vi "Mcp2210 Request Spi Bus Rel.vi"(8 "error in (no error)":errorcluster, 10 "SPI Release ACK Pin Define":u8, 11 "handle":i32) -> (0 "error out":errorcluster, 3 "handle out":i32)   [LabVIEW 2015, in "mcp2210.lvlib"]
doc: "Request the release of the SPI bus and set the value of the \"SPI Bus Release ACK\" pin\nif GP7 is assigned to this dedicated function and if the bus can be released.\nIf SPI transfer is in progress, the bus is not released, the command returns M_E_ERR_SPI_XFER_ONGOING\nerrorcode and the host application should either wait the transfer completion or cancel it\n(by using M_Mcp2210_CancelSpiTxfer) and request again the SPI bus release.\nParameters:\nInputs:\n- IntPtr handle - The device handle. Cannot be NULL.\n- unsigned char ackPinVal - the value of the \"SPI Bus Release ACK\" pin if the\ncommand succeeds and the GP7 is assigned to alternate function 2.\nOutputs:\n- none\nReturns:\n- 0 for success: M_E_SUCCESS\n- negative error code: M_E_ERR_NULL, M_E_ERR_INVALID_HANDLE_VALUE, M_E_ERR_INVALID_PARAMETER\nM_E_ERR_UNKOWN_ERROR\nM_E_ERR_HID_TIMEOUT, M_E_ERR_HID_RW_FILEIO\nM_E_ERR_CMD_ECHO, M_E_ERR_CMD_FAILED\nM_E_ERR_SPI_XFER_ONGOING\n\nMCP2210_DLL_UM_API int __stdcall Mcp2210_RequestSpiBusRel(void *handle, unsigned char ackPinVal);"
uses:
  <userlib>/mcp2210/mcp2210.lvlib
  <userlib>/mcp2210/mcp2210_dll_um_x86.dll
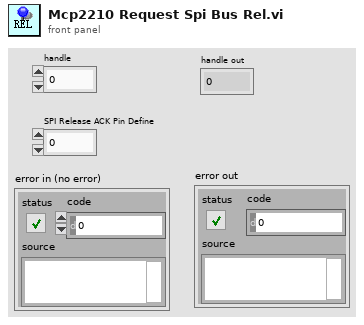
[diagram p1: front panel]
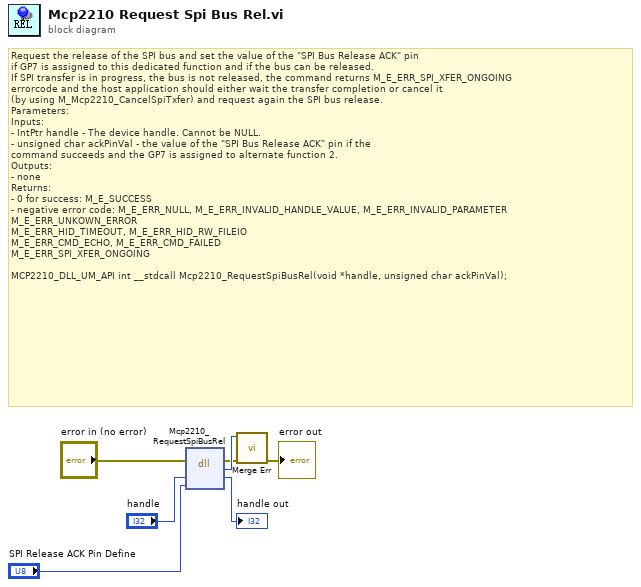
[diagram p0: block diagram]
diagram:
  # "Request the release of the SPI bus and set the value of the \"SPI Bus Release ACK\" pin\nif GP7 is assigned to this dedicated function and if the bus can be released.\nIf SPI transfer is in progress, the bus is not released, the command returns M_E_ERR_SPI_XFER_ONGOING\nerrorcode and the host application should either wait the transfer completion or cancel it\n(by using M_Mcp2210_CancelSpiTxfer) and request again the SPI bus release.\nParameters:\nInputs:\n- IntPtr handle - The device handle. Cannot be NULL.\n- unsigned char ackPinVal - the value of the \"SPI Bus Release ACK\" pin if the\ncommand succeeds and the GP7 is assigned to alternate function 2.\nOutputs:\n- none\nReturns:\n- 0 for success: M_E_SUCCESS\n- negative error code: M_E_ERR_NULL, M_E_ERR_INVALID_HANDLE_VALUE, M_E_ERR_INVALID_PARAMETER\nM_E_ERR_UNKOWN_ERROR\nM_E_ERR_HID_TIMEOUT, M_E_ERR_HID_RW_FILEIO\nM_E_ERR_CMD_ECHO, M_E_ERR_CMD_FAILED\nM_E_ERR_SPI_XFER_ONGOING\n\nMCP2210_DLL_UM_API int __stdcall Mcp2210_RequestSpiBusRel(void *handle, unsigned char ackPinVal);"
  n1 = dll-call lib="D:/LabVIEW 2015/user.lib/mcp2210/mcp2210_dll_um_x86.*" fn="Mcp2210_RequestSpiBusRel"(error in="error in (no error)", "handle"="handle", "ackPinVal"="SPI Release ACK Pin Define") -> (error out=w3:errorcluster, "return type"=w4:i32, "handle"=→"handle out":i32)  [unwired: 3 in, 1 out]
  n2 = call <userlib>:"Merge Err.vi"("error in (no error)"=w3, "return type"=w4) -> ("error out"=→"error out":errorcluster)  [unwired: 9 in]
